vi "Start_Popup.vi"(0 "Application_Directory":path, 11 "Error_In":errorcluster) -> (15 "Error_Out":errorcluster)   [LabVIEW 2023]
doc: "This is a VI work as one of the front panel of the Game, asking the user to start the game."
uses:
  Controls/Bool_Button.ctl
  Controls/State.ctl
panel:
  in  "Close?":T1
  in  "Start?":T1
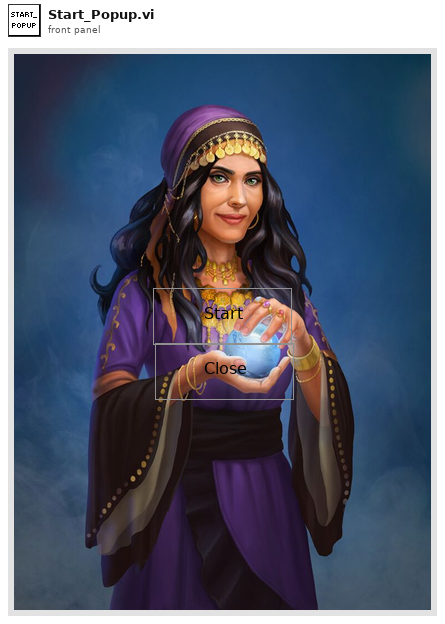
[diagram p1: front panel]
types:
  T1 = typedef "Bool_Button.ctl" = bool
  T2 = enum32{"Invalid", "Standard", "Closed", "Hidden", "Minimized", "Maximized"}
  T3 = typedef "State.ctl" = enum16{"Close", "Password_Popup", "Start_Popup", "Wizard_Msg", "Get_Name_DoB", "Lucky_Number", "Q-1", "Q-2", "Q-3", "Nature_of_the_Person"}
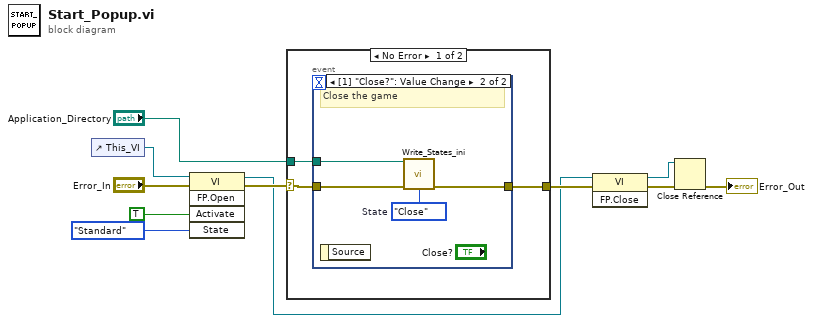
[diagram p0: block diagram]
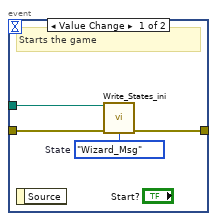
[diagram p2: hidden frame]
diagram:
  n1 = control-ref of="This_VI"() -> (w3:refnum<vi>)
  n2 = invoke class="VI" method="FP.Open"(reference=w3, error in="Error_In", "Activate"=TRUE ("Activate?"), "State"=T2."Standard") -> (reference out=w4:refnum<vi>, error out=w9:errorcluster)  [unwired: 1 in, 3 out]
  n3 = case shown="No Error" w9 {
    selector: w9 -> [w14 w23]
    tunnel: [w13 w23] -> w10
    tunnel: "Application_Directory" -> [w12 _]
    frame No Error {
      n4 = event shown="[1] \"Close?\": Value Change" {
        selector: _ -> [_ _]
        dyn-events: _ -> [_ _]
        timeout: _ -> [_ _]
        tunnel: w14 -> [w18 w22]
        tunnel: [w17 w21] -> w13
        tunnel: w12 -> [w15 w19]
        event Value Change {
          w16 = State."Wizard_Msg"  # State
          # "Starts the game"
          n5 = event-data() -> ()  [unwired: 1 in, 1 out]
          n6 = call "Write_States_ini.vi"("Application_Directory"=w15, "Error_In"=w18, "State"=w16) -> ("Error_Out"=w17:errorcluster)  [unwired: 12 in]
        }
        event Value Change {
          w20 = State."Close"  # State
          # "Close the game"
          n7 = event-data() -> ()  [unwired: 1 in, 1 out]
          n8 = call "Write_States_ini.vi"("Application_Directory"=w19, "Error_In"=w22, "State"=w20) -> ("Error_Out"=w21:errorcluster)  [unwired: 12 in]
        }
      }
    }
    frame Error {
    }
  }
  n9 = invoke class="VI" method="FP.Close"(reference=w4, error in=w10) -> (reference out=w5:refnum<vi>, error out=w7:errorcluster)  [unwired: 1 in, 1 out]
  n10 = Close Reference(reference=w5, error in (no error)=w7) -> (error out=→"Error_Out":errorcluster)
